vi "Expo.vi"(1 "Numeric":i32) -> (0 "Array":i32[](array[numeric]))   [LabVIEW 2014]
uses:
  wlmData.dll
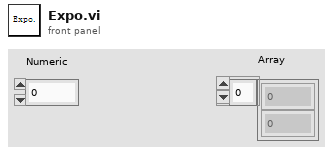
[diagram p1: front panel]
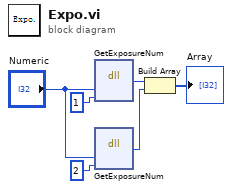
[diagram p0: block diagram]
diagram:
  n1 = dll-call lib="wlmData.dll" fn="GetExposureNum"("num"="Numeric", "arr"=1) -> ("res"=w2:i32)  [unwired: 5 in, 2 out]
  n2 = dll-call lib="wlmData.dll" fn="GetExposureNum"("num"="Numeric", "arr"=2) -> ("res"=w1:i32)  [unwired: 5 in, 2 out]
  n3 = Build Array(w2, w1) -> (→"Array":i32[])
